vi "Get All Commits.vi"(8 "error in":errorcluster, 11 "Peer Review in":refnum<class "Peer Review.lvclass">) -> (0 "error out":errorcluster, 3 "Peer Review out":refnum<class "Peer Review.lvclass">)   [LabVIEW 2020, in "Peer Review.lvclass"]
uses:
  Peer Review.lvclass
  Peer Review.lvclass/Peer Review.ctl
  <vilib>/Utility/error.llb/Trim Whitespace One-Sided.vi
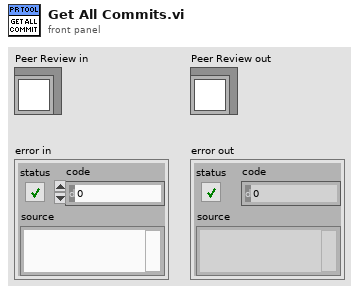
[diagram p1: front panel]
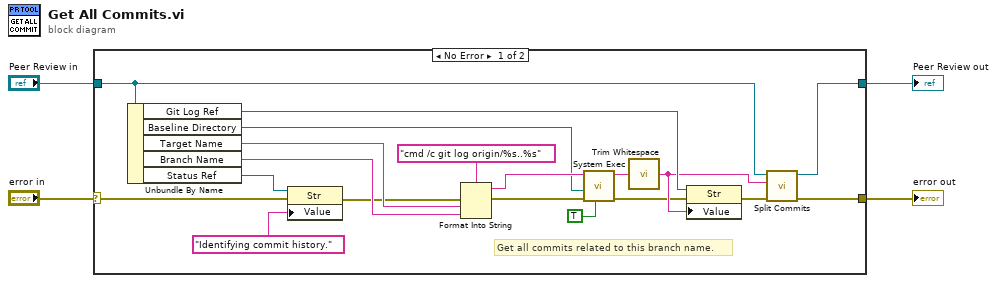
[diagram p0: block diagram]
diagram:
  n1 = case shown="No Error" "error in" {
    selector: "error in" -> [w7 w25]
    tunnel: "Peer Review in" -> [w22 w24]
    tunnel: [w17 w24] -> w2
    tunnel: [w16 w25] -> w1
    frame No Error {
      # "Get all commits related to this branch name."
      n2 = Unbundle By Name(w22) -> ("Git Log Ref"=w23:refnum<vi>, "Baseline Directory"=w11:path, "Target Name"=w10:string, "Branch Name"=w9:string, "Status Ref"=w8:refnum<vi>)
      n3 = property on="Property Node" class="Str"(reference=w8, error in=w7, "Value"="Identifying commit history.") -> (error out=w6:errorcluster)  [unwired: 1 out]
      n4 = Format Into String(format string="cmd /c git log origin/%s..%s" ("String 2"), error in=w6, w10, w9) -> (resulting string=w14:string, error out=w12:errorcluster)  [unwired: 1 in]
      n5 = call <vilib>:"System Exec.vi"("run minimized? (F)"=TRUE, "error in (no error)"=w12, "working directory"=w11, "command line"=w14) -> ("error out"=w18:errorcluster, "standard output"=w20:string)  [unwired: 4 in, 2 out]
      n6 = call <vilib>:"Trim Whitespace.vi"("string"=w20) -> ("trimmed string"=w21:string)  [unwired: 1 in]
      n7 = property on="Property Node" class="Str"(reference=w23, error in=w18, "Value"=w21) -> (error out=w19:errorcluster)  [unwired: 1 out]
      n8 = call "Split Commits.vi"("error in"=w19, "Commit String"=w21, "Peer Review in"=w22) -> ("error out"=w16:errorcluster, "Peer Review out"=w17:refnum<class "Peer Review.lvclass">)  [unwired: 7 in]
    }
    frame Error {
    }
  }
  "Peer Review out" <- w2
  "error out" <- w1
